vi "HTS_INJECT_WELL.vi"(4 "Final Flush?":bool=TRUE, 6 "Inject all wells?":bool=TRUE, 7 "Loader Settings":T1={"Sample Flow Rate (uL/s)"=1.0, "Sample Volume (uL)"=4.0, "Mixing Volume (uL)"=30, "Mixing Speed (uL/s)"=100, "Mix#"=2, "Wash Volume (uL)"=200, "INJECTION_MODE"=enum."HT"} {"Sample Volume (uL)" min=2.0 max=200.0 step=0.5; "Mixing Volume (uL)" min=5 max=100 step=5; "Mixing Speed (uL/s)" min=25 max=250 step=5; "Sample Flow Rate (uL/s)" min=0.5 max=3.0 step=0.5 format="%_2f"; "Mix#" min=0 max=5 step=1; "Wash Volume (uL)" min=200 max=800 step=20}, 8 "Error IN":errorcluster, 9 "INJECTION_MODE":T2=enum."HT", 10 "Wells to Inject":T3[](array[typedef])=[{"Column"=enum."1", "Row"=enum."A"}, {"Column"=enum."2", "Row"=enum."A"}, {"Column"=enum."3", "Row"=enum."A"}, {"Column"=enum."4", "Row"=enum."A"}], 11 "VISA resource IN":refnum<visa-resource-name>="HTS") -> (0 "Error OUT":errorcluster, 1 "Acq. time(s)":dbl=15.448000431060791, 3 "VISA resource OUT":refnum<visa-resource-name>="HTS")   [LabVIEW 2009]
uses:
  HTS_WELL.ctl
  HTS_COLUMN.ctl
  HTS_ROW.ctl
  HTS_INJECTION_MODE.ctl
  HTS_LOADER_SETTINGS.ctl
  GA_GLOBAL_VARIABLES.vi
  EVENT_ORIGIN.ctl
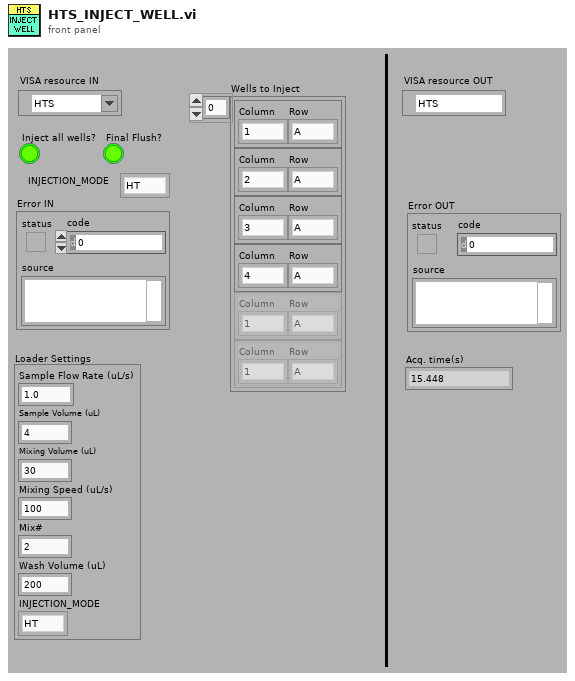
[diagram p1: front panel]
types:
  T1 = typedef "HTS_LOADER_SETTINGS.ctl" = cluster{"Sample Flow Rate (uL/s)":dbl, "Sample Volume (uL)":dbl, "Mixing Volume (uL)":i32, "Mixing Speed (uL/s)":i32, "Mix#":i32, "Wash Volume (uL)":i32, "INJECTION_MODE":T2}
  T2 = typedef "HTS_INJECTION_MODE.ctl" = enum16{"STD", "HT"}
  T3 = typedef "HTS_WELL.ctl" = cluster{"Column":T4, "Row":T5}
  T4 = typedef "HTS_COLUMN.ctl" = enum16{"1", "2", "3", "4", "5", "6", "7", "8", "9", "10", "11", "12"}
  T5 = typedef "HTS_ROW.ctl" = enum16{"A", "B", "C", "D", "E", "F", "G", "H"}
  T6 = typedef "EVENT_ORIGIN.ctl" = enum16{"GLOBAL", "HTS", "MULTIMEK", "CRANE", "SHAKER", "SNIFFER"}
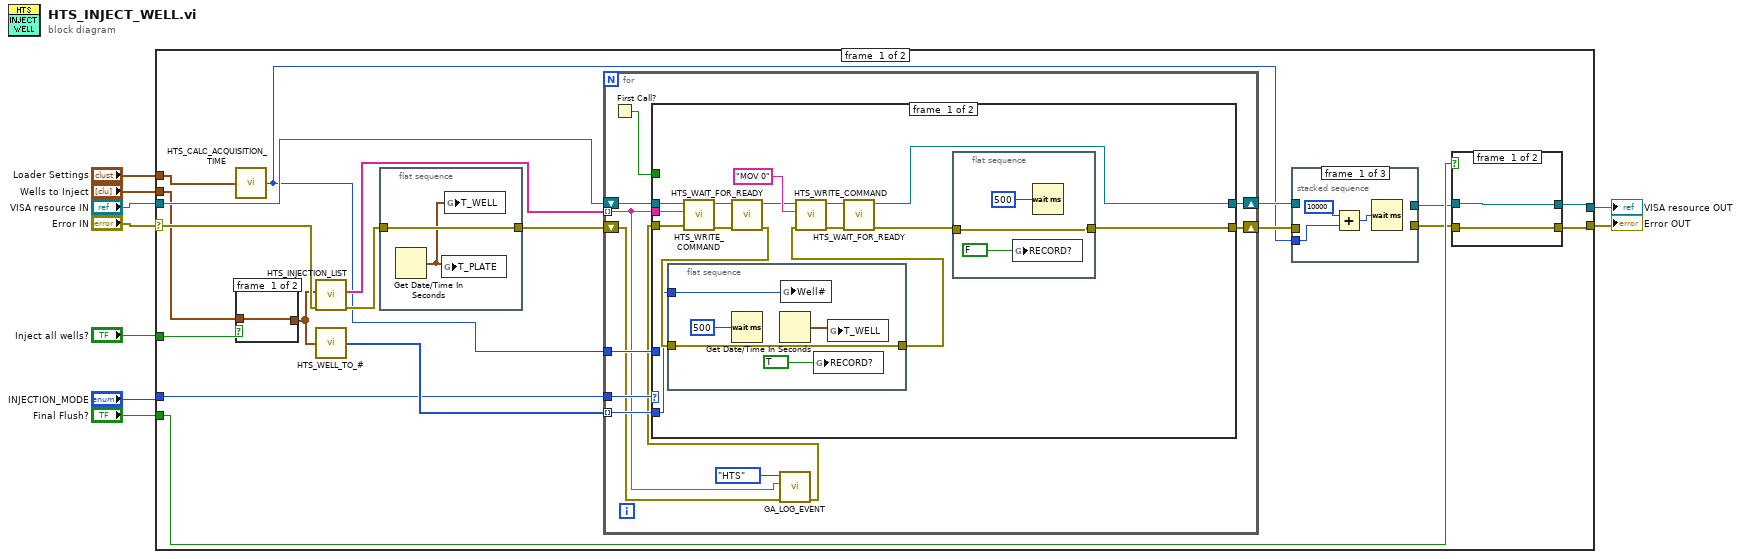
[diagram p0: block diagram]
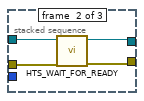
[diagram p2: hidden frame]
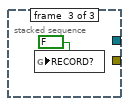
[diagram p3: hidden frame]
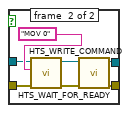
[diagram p4: hidden frame]
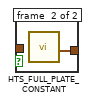
[diagram p5: hidden frame]
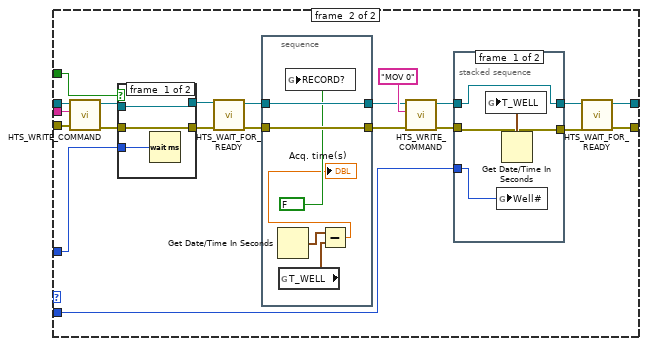
[diagram p6: hidden frame]
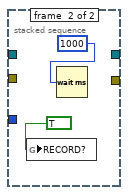
[diagram p7: hidden frame]
diagram:
  n1 = case shown="No Error" "Error IN" {
    selector: "Error IN" -> [w27 w123]
    tunnel: [w23 w123] -> w9
    tunnel: [w22 w122] -> w8
    tunnel: "VISA resource IN" -> [w28 w122]
    tunnel: "Wells to Inject" -> [w25 _]
    tunnel: "Inject all wells?" -> [w24 _]
    tunnel: "Final Flush?" -> [w21 _]
    tunnel: "INJECTION_MODE" -> [w16 _]
    tunnel: "Loader Settings" -> [w15 _]
    frame #0 {
      n2 = call "HTS_CALC_ACQUISITION_TIME.vi"("Loader Settings"=w15) -> ("Numeric"=w12:u32)
      n3 = case shown="True" w24 {
        tunnel: [w48 w49] -> w20
        tunnel: w25 -> [w48 _]
        frame #0 {
        }
        frame #1 {
          n4 = call "HTS_FULL_PLATE_CONSTANT.vi"() -> ("Array"=w49:T3[])
        }
      }
      n5 = call "HTS_INJECTION_LIST.vi"("Error IN"=w27, "Wells  to inject (Well array)"=w20) -> ("Error OUT"=w18:errorcluster, "Commands (String Array)"=w26:string[])  [unwired: 8 out]
      n6 = call "HTS_WELL_TO_#.vi"("Well Array"=w20) -> ("Position Array"=w19:i32[])
      n7 = flat-sequence {
        tunnel: w18 -> [w38]
        tunnel: [w38] -> w17
        frame #0 {
          n8 = Get Date/Time In Seconds() -> (seconds since 1Jan1904=w37:timestamp)
          n9 = global write "GA_GLOBAL_VARIABLES.vi" "T_PLATE"(w37) -> ()
          n10 = global write "GA_GLOBAL_VARIABLES.vi" "T_WELL"(w37) -> ()
        }
      }
      n11 = for {
        tunnel: w26 -> [w51] mode=indexing
        shift-right: [w58] -> w13
        shift-left: w17 -> [w53]
        shift-right: [w60] -> w14
        shift-left: w28 -> [w59]
        tunnel: w19 -> [w57] mode=indexing
        tunnel: w16 -> [w56]
        tunnel: w12 -> [w54]
        n12 = First Call?() -> (First Call?: T/F=w55:bool)
        n13 = call "GA_LOG_EVENT.vi"("error in"=w53, "Event description"=w51, "Event Origin"=EVENT_ORIGIN."HTS") -> ("error out"=w52:errorcluster)  [unwired: 8 out]
        n14 = case shown="\"HT\"" w56 {
          tunnel: [w75 w85] -> w60
          tunnel: w59 -> [w73 w103]
          tunnel: w51 -> [w72 w102]
          tunnel: w52 -> [w66 w104]
          tunnel: [w62 w84] -> w58
          tunnel: w57 -> [w61 w100]
          tunnel: w55 -> [_ w97]
          tunnel: w54 -> [_ w96]
          frame #0 {
            n15 = flat-sequence {
              tunnel: w65 -> [w82]
              tunnel: [w82] -> w64
              tunnel: w61 -> [w80]
              frame #0 {
                n16 = Wait (ms)(milliseconds to wait=u32 500) -> ()  [unwired: 1 out]
                n17 = Get Date/Time In Seconds() -> (seconds since 1Jan1904=w83:timestamp)
                n18 = global write "GA_GLOBAL_VARIABLES.vi" "Well#"(w80) -> ()
                n19 = global write "GA_GLOBAL_VARIABLES.vi" "RECORD?"(TRUE ("INJECTING?")) -> ()
                n20 = global write "GA_GLOBAL_VARIABLES.vi" "T_WELL"(w83) -> ()
              }
            }
            n21 = call "HTS_WRITE_COMMAND.vi"("Error IN"=w66, "Command"=w72, "VISA resource IN"=w73) -> ("Error OUT"=w67:errorcluster, "VISA resource OUT"=w68:refnum<visa-resource-name>)  [unwired: 7 out]
            n22 = call "HTS_WAIT_FOR_READY.vi"("Error IN"=w67, "VISA resource IN"=w68) -> ("Error OUT"=w65:errorcluster, "VISA resource OUT"=w70:refnum<visa-resource-name>)  [unwired: 1 in, 7 out]
            n23 = call "HTS_WRITE_COMMAND.vi"("Error IN"=w64, "Command"="MOV 0", "VISA resource IN"=w70) -> ("Error OUT"=w74:errorcluster, "VISA resource OUT"=w69:refnum<visa-resource-name>)  [unwired: 7 out]
            n24 = call "HTS_WAIT_FOR_READY.vi"("Error IN"=w74, "VISA resource IN"=w69) -> ("Error OUT"=w63:errorcluster, "VISA resource OUT"=w75:refnum<visa-resource-name>)  [unwired: 1 in, 7 out]
            n25 = flat-sequence {
              tunnel: w63 -> [w78]
              tunnel: [w78] -> w62
              frame #0 {
                n26 = global write "GA_GLOBAL_VARIABLES.vi" "RECORD?"(FALSE ("INJECTING?")) -> ()
                n27 = Wait (ms)(milliseconds to wait=u32 500) -> ()  [unwired: 1 out]
              }
            }
          }
          frame #1 {
            n28 = call "HTS_WRITE_COMMAND.vi"("Error IN"=w104, "Command"=w102, "VISA resource IN"=w103) -> ("Error OUT"=w94:errorcluster, "VISA resource OUT"=w95:refnum<visa-resource-name>)  [unwired: 7 out]
            n29 = case shown="False" w97 {
              tunnel: w95 -> [w113 w115]
              tunnel: [w113 w115] -> w90
              tunnel: w94 -> [w112 w114]
              tunnel: [w112 w114] -> w93
              tunnel: w96 -> [w111 _]
              frame #0 {
                n30 = Wait (ms)(milliseconds to wait=w111) -> ()  [unwired: 1 out]
              }
              frame #1 {
              }
            }
            n31 = call "HTS_WAIT_FOR_READY.vi"("Error IN"=w93, "VISA resource IN"=w90) -> ("Error OUT"=w92:errorcluster, "VISA resource OUT"=w91:refnum<visa-resource-name>)  [unwired: 1 in, 7 out]
            n32 = stacked-sequence {
              tunnel: w91 -> [w121]
              tunnel: [w121] -> w99
              tunnel: w92 -> [w120]
              tunnel: [w120] -> w98
              frame #0 {
                n33 = Get Date/Time In Seconds() -> (seconds since 1Jan1904=w118:timestamp)
                n34 = global read "GA_GLOBAL_VARIABLES.vi" "T_WELL"() -> (w117:timestamp)
                n35 = global write "GA_GLOBAL_VARIABLES.vi" "RECORD?"(FALSE ("INJECTING?")) -> ()
                n36 = Subtract(x=w118, y=w117) -> (x-y=→"Acq. time(s)":dbl)
              }
            }
            n37 = call "HTS_WRITE_COMMAND.vi"("Error IN"=w98, "Command"="MOV 0", "VISA resource IN"=w99) -> ("Error OUT"=w88:errorcluster, "VISA resource OUT"=w89:refnum<visa-resource-name>)  [unwired: 7 out]
            n38 = stacked-sequence {
              tunnel: [w106 _] -> w87
              tunnel: w100 -> [w107 _]
              tunnel: w88 -> [w106 _]
              tunnel: w89 -> [w105 _]
              tunnel: [w105 _] -> w86
              frame #0 {
                n39 = global write "GA_GLOBAL_VARIABLES.vi" "Well#"(w107) -> ()
                n40 = Get Date/Time In Seconds() -> (seconds since 1Jan1904=w108:timestamp)
                n41 = global write "GA_GLOBAL_VARIABLES.vi" "T_WELL"(w108) -> ()
              }
              frame #1 {
                n42 = global write "GA_GLOBAL_VARIABLES.vi" "RECORD?"(TRUE ("INJECTING?")) -> ()
                n43 = Wait (ms)(milliseconds to wait=u32 1000) -> ()  [unwired: 1 out]
              }
            }
            n44 = call "HTS_WAIT_FOR_READY.vi"("Error IN"=w87, "VISA resource IN"=w86) -> ("Error OUT"=w84:errorcluster, "VISA resource OUT"=w85:refnum<visa-resource-name>)  [unwired: 1 in, 7 out]
          }
        }
      }
      n45 = stacked-sequence {
        tunnel: w14 -> [_ w35 _]
        tunnel: w13 -> [_ w34 _]
        tunnel: w12 -> [w30 _ _]
        tunnel: [_ w33 _] -> w11
        tunnel: [_ w32 _] -> w10
        frame #0 {
          n46 = Add(x=u32 10000, y=w30) -> (x+y=w29:u32)
          n47 = Wait (ms)(milliseconds to wait=w29) -> ()  [unwired: 1 out]
        }
        frame #1 {
          n48 = call "HTS_WAIT_FOR_READY.vi"("Error IN"=w34, "VISA resource IN"=w35) -> ("Error OUT"=w33:errorcluster, "VISA resource OUT"=w32:refnum<visa-resource-name>)  [unwired: 1 in, 7 out]
        }
        frame #2 {
          n49 = global write "GA_GLOBAL_VARIABLES.vi" "RECORD?"(FALSE ("INJECTING?")) -> ()
        }
      }
      n50 = case shown="True" w21 {
        tunnel: [w39 w44] -> w23
        tunnel: [w40 w43] -> w22
        tunnel: w10 -> [w40 w42]
        tunnel: w11 -> [w39 w41]
        frame #0 {
        }
        frame #1 {
          n51 = call "HTS_WRITE_COMMAND.vi"("Error IN"=w41, "Command"="MOV 0", "VISA resource IN"=w42) -> ("Error OUT"=w46:errorcluster, "VISA resource OUT"=w45:refnum<visa-resource-name>)  [unwired: 7 out]
          n52 = call "HTS_WAIT_FOR_READY.vi"("Error IN"=w46, "VISA resource IN"=w45) -> ("Error OUT"=w44:errorcluster, "VISA resource OUT"=w43:refnum<visa-resource-name>)  [unwired: 1 in, 7 out]
        }
      }
    }
    frame #1 {
    }
  }
  "Error OUT" <- w9
  "VISA resource OUT" <- w8
